vi "Main.vi"(11 "Module Admin":refnum<class "Delacor_lib_QMH_Cloneable Module Admin.lvclass">) -> ()   [LabVIEW 2020, in "TCP_Client.lvlib"]
doc: "This template is based off of the Queued Message Handler design pattern and the Queued Message Handler project template that ships with LabVIEW.\n\nThe main difference is that the queue is private to this module and communication between modules is performed via Broadcast and Request events.\n\nRequest events are wrapped in public API methods and are handled in the Event Handling Loop (EHL) of this VI. Any module can register for Broadcast events sent by this module. The EHL generates messages based on user interface actions.\n\nThe Message Handling Loop (MHL) processes messages generated by the EHL, or by other messages. The messages are string values, so new messages can be added easily to the Message Cases case structure in the MHL. Each message cluster can also provide an optional value for Message Data, which is a variant that can be converted to whatever message-specific data is required.\n_____\nBased on DQMH Project Template 6.0.0.91."
uses:
  TCP_Client.lvlib
  <vilib>/Delacor/Delacor QMH/Libraries/Cloneable Module Admin_class/Delacor_lib_QMH_Cloneable Module Admin.lvclass
  C:/Program Files (x86)/National Instruments/LabVIEW 2020/vi.lib/Delacor/Delacor QMH/Libraries/Module Admin_class/Delacor_lib_QMH_Module Admin.lvclass
  Module Data--cluster.ctl
  <vilib>/Delacor/Delacor QMH/Libraries/Cloneable Module Admin_class/Delacor_lib_QMH_Cloneable Module Admin.lvclass/Delacor_lib_QMH_Cloneable Module Admin.ctl
  <vilib>/Delacor/Delacor QMH/Libraries/Message Queue_class/Delacor_lib_QMH_Message Queue.lvclass/Delacor_lib_QMH_Message Queue.ctl
  Stop Argument--cluster.ctl
  <vilib>/Delacor/Delacor QMH/Libraries/Module Admin_class/Delacor_lib_QMH_Module Admin.lvclass/Delacor_lib_QMH_Module Admin.ctl
  <vilib>/Utility/miscctls.llb/LVPointTypeDef.ctl
  <vilib>/Delacor/Delacor QMH/Libraries/Cloneable Module Admin_class/Delacor_lib_QMH_Get Module ID.vi
  <vilib>/Delacor/Delacor QMH/Libraries/Message Queue_class/Delacor_lib_QMH_Enqueue Message (Single).vi
  <vilib>/Delacor/Delacor QMH/Libraries/Module Admin_class/Delacor_lib_QMH_Get External Launch.vi
  <vilib>/Utility/error.llb/Error Cluster From Error Code.vi
  <vilib>/ErrorRing/Error Ring.xnode
  <vilib>/Delacor/Delacor QMH/Libraries/Message Queue_class/Delacor_lib_QMH_Message Queue.lvclass
  TCP_Server/TCP_Server.lvlib
panel:
  out "Module ID":i32=-1
  out "Receive":T1 {"Horizontal Pointer Slide" scale=0.0..10.0; "Gauge" scale=0.0..10.0}
  out "Data from Server":dbl(graph)
  out "error out":errorcluster
  out "Status":string
  in  "Simulate EHL Error":bool
  in  "Simulate MHL Error":bool
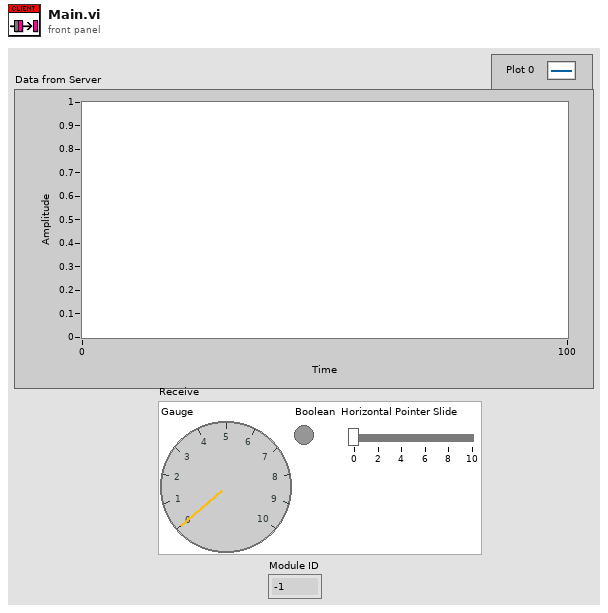
[diagram p1: front panel]
types:
  T1 = cluster{"Gauge":dbl, "Boolean":bool, "Horizontal Pointer Slide":i32}
  T2 = typedef "TCP_Client.lvlib/Request Events--cluster.ctl" = cluster{"Stop Module":refnum<user-event>, "Show Panel":refnum<user-event>, "Hide Panel":refnum<user-event>, "Show Diagram":refnum<user-event>, "Get Module Execution Status":refnum<user-event>, "Connect TCP to Server":refnum<user-event>, "CheckClientSelection":refnum<user-event>, "AllSelection":refnum<user-event>}
  T3 = typedef "TCP_Server.lvlib/Broadcast Events--cluster.ctl" = cluster{"Module Did Init":refnum<user-event>, "Status Updated":refnum<user-event>, "Error Reported":refnum<user-event>, "Module Did Stop":refnum<user-event>, "Update Module Execution Status":refnum<user-event>, "ClientSelect":refnum<user-event>, "SelectAll":refnum<user-event>}
  T4 = typedef "TCP_Client.lvlib/Module Data--cluster.ctl" = cluster{"Status":string}
  T5 = cluster{"Gauge":dbl, "Boolean":bool, "Horizontal Pointer Slide":dbl}
  T6 = enum32{"invalid lock state", "Not Locked", "Locked (No Password)", "Password-protected"}
  T7 = typedef "TCP_Client.lvlib/Stop Argument--cluster.ctl" = cluster{"Module ID":i32, "Origin":string, "Exit via Stop Module Req?":bool, "Wait for Module to stop?":bool}
  T8 = typedef "LVPointTypeDef.ctl" = cluster{"Horizontal":i16, "Vertical":i16}
  T9 = enum32{"Invalid", "Standard", "Closed", "Hidden", "Minimized", "Maximized"}
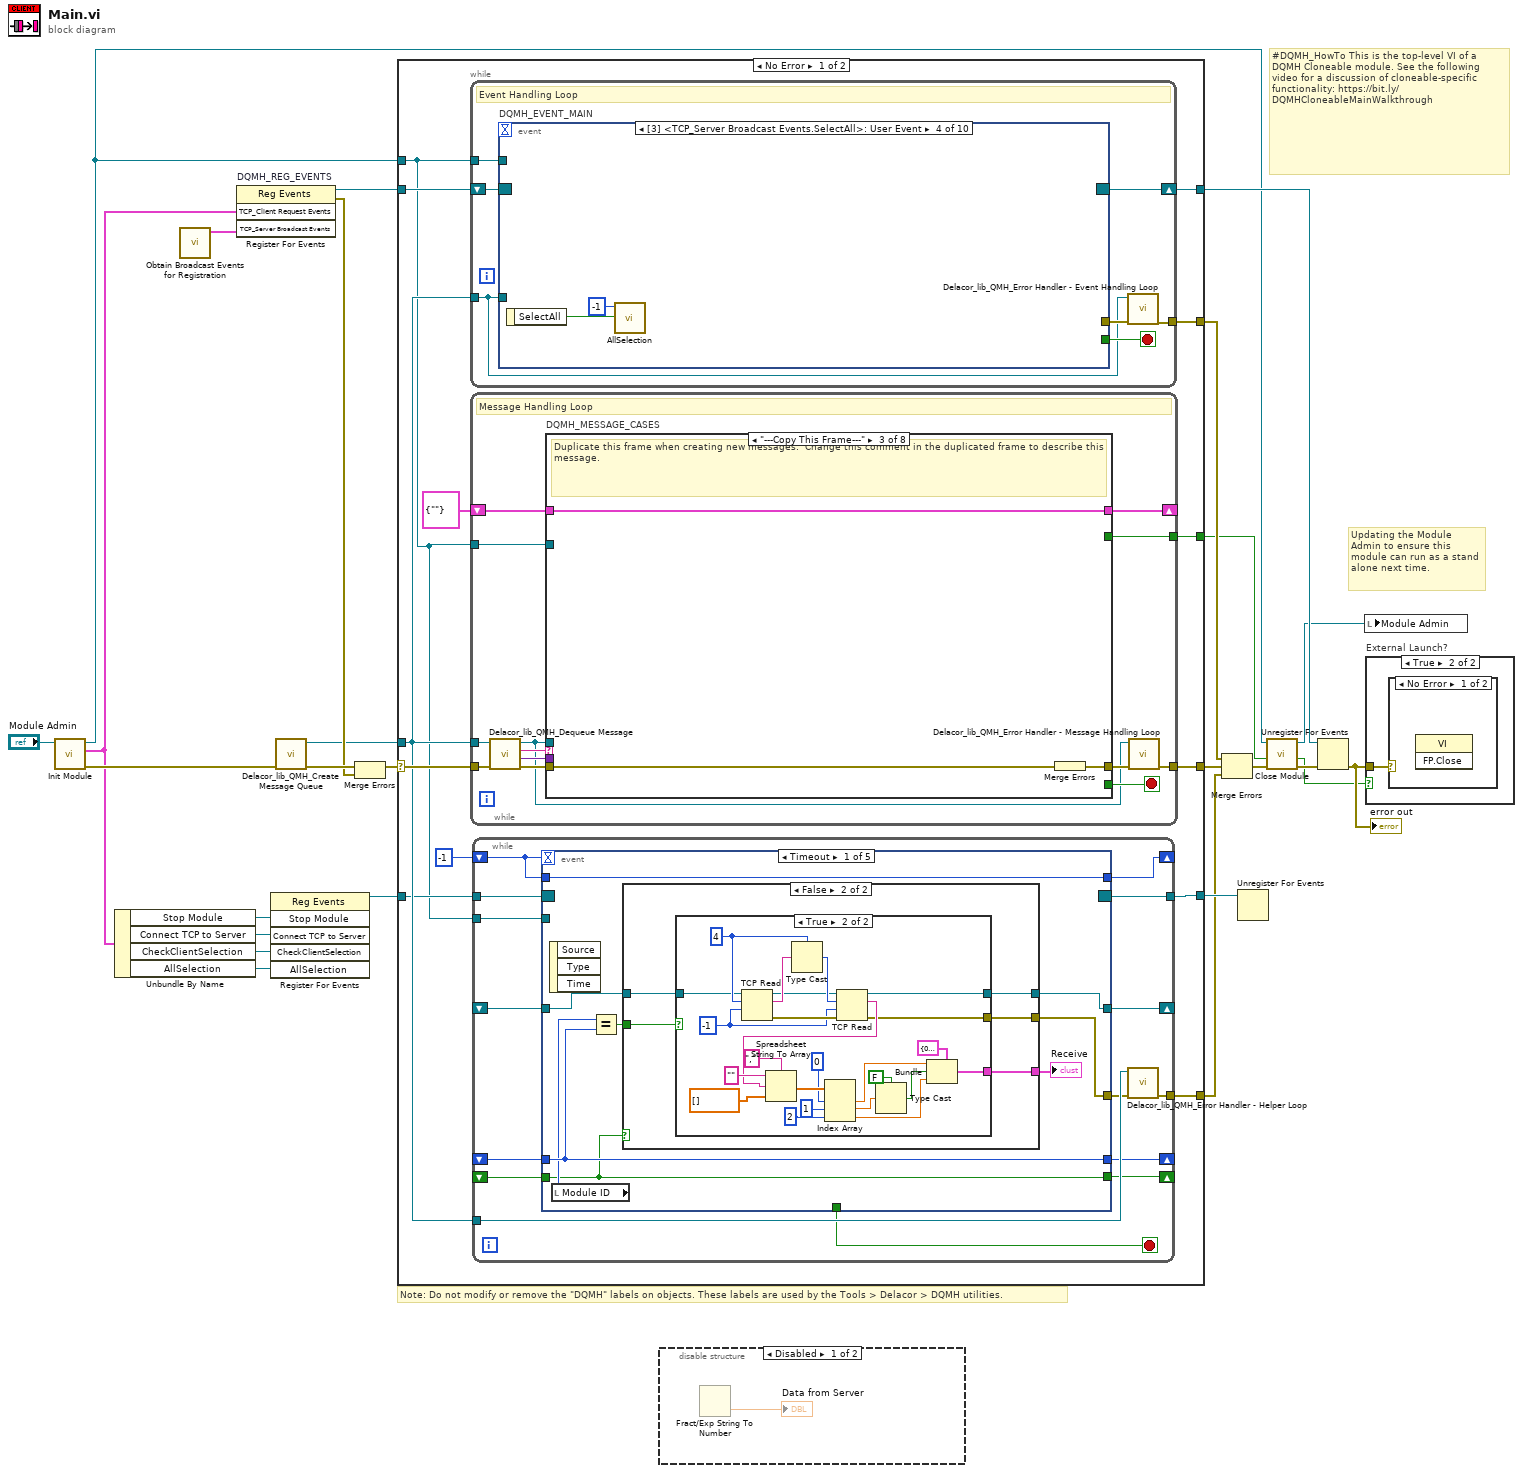
[diagram p0: block diagram]
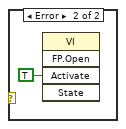
[diagram p4: hidden frame]
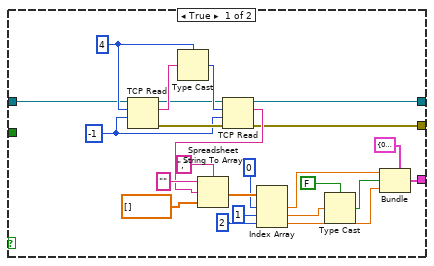
[diagram p5: hidden frame]
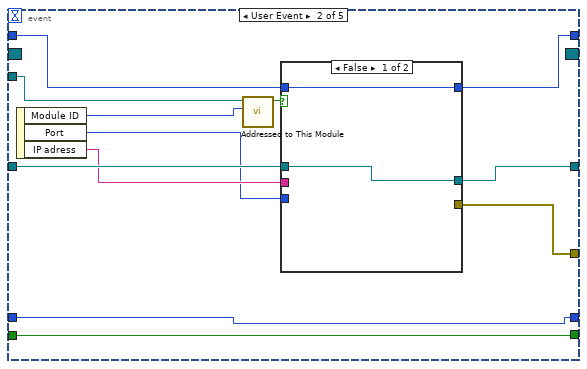
[diagram p7: hidden frame]
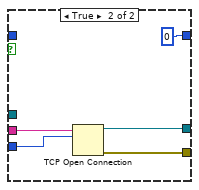
[diagram p8: hidden frame]
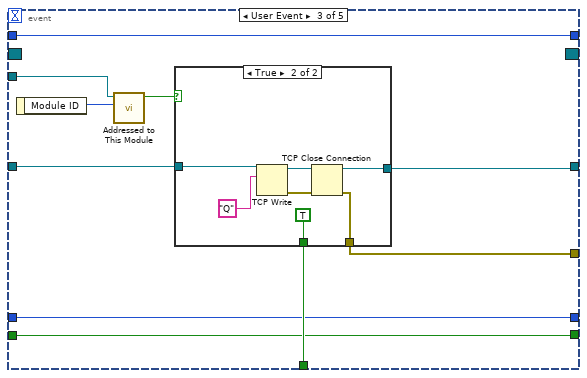
[diagram p9: hidden frame]
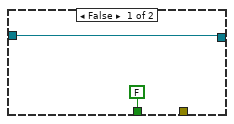
[diagram p10: hidden frame]
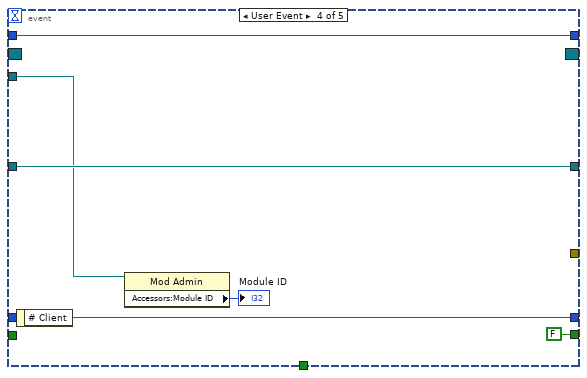
[diagram p11: hidden frame]
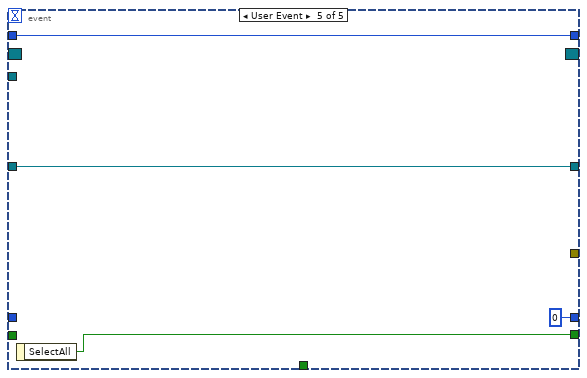
[diagram p12: hidden frame]
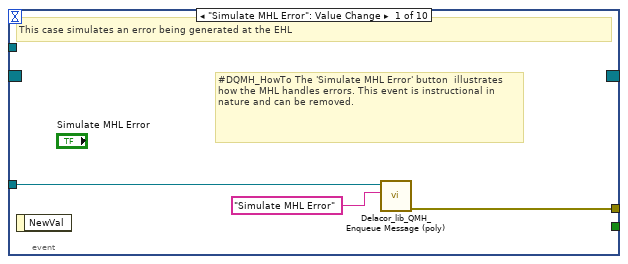
[diagram p13: hidden frame]
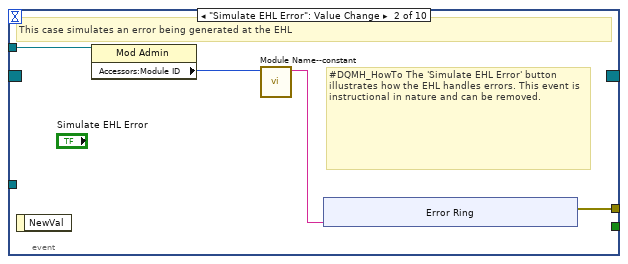
[diagram p14: hidden frame]
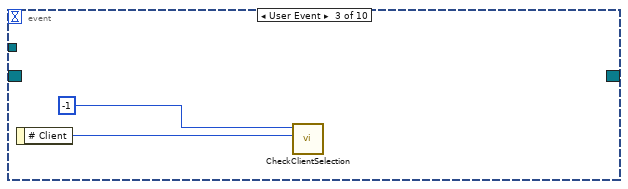
[diagram p15: hidden frame]
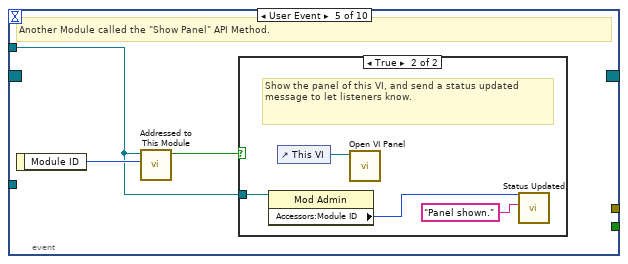
[diagram p16: hidden frame]
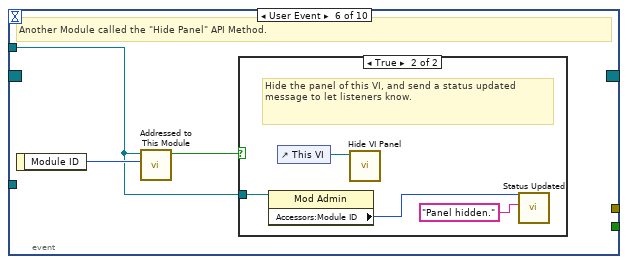
[diagram p18: hidden frame]
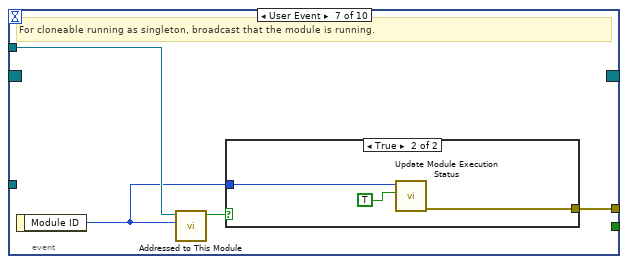
[diagram p20: hidden frame]
diagram:
  # "#DQMH_HowTo This is the top-level VI of a DQMH Cloneable module. See the following video for a discussion of cloneable-specific functionality: https://bit.ly/DQMHCloneableMainWalkthrough"
  # "Note: Do not modify or remove the \"DQMH\" labels on objects. These labels are used by the Tools > Delacor > DQMH utilities."
  # "Updating the Module Admin to ensure this module can run as a stand alone next time."
  n1 = call "Init Module.vi"("Cloneable Module Admin in"="Module Admin") -> ("error out"=w23:errorcluster, "TCP_Client Request Events"=w7:T2, "Cloneable Module Admin out"=w13:refnum<class "Delacor_lib_QMH_Cloneable Module Admin.lvclass">)  [unwired: 8 in]
  n2 = Unbundle By Name(w7) -> ("Stop Module"=w6:refnum<user-event>, "Connect TCP to Server"=w4:refnum<user-event>, "CheckClientSelection"=w2:refnum<user-event>, "AllSelection"=w1:refnum<user-event>)
  n3 = call "Obtain Broadcast Events for Registration.vi"() -> ("TCP_Server Broadcast Events"=w3:T3)  [unwired: 9 in, 2 out]
  n4 = register-events "DQMH_REG_EVENTS"(w7, w3) -> (reference out=w16:refnum<event-registration>, error out=w18:errorcluster)  [unwired: 2 in]
  n5 = register-events(w6, w4, w2, w1) -> (reference out=w5:refnum<event-registration>)  [unwired: 2 in, 1 out]
  n6 = call <vilib>:"Delacor_lib_QMH_Create Message Queue.vi"("error in"=w23) -> ("error out"=w20:errorcluster, "Message Queue"=w15:refnum<class "Delacor_lib_QMH_Message Queue.lvclass">)  [unwired: 9 in]
  n7 = Merge Errors(w20, w18) -> (w19:errorcluster)
  n8 = case shown="No Error" w19 {
    selector: w19 -> [w37 w365]
    tunnel: [w39 w364] -> w24
    tunnel: [w36 w372] -> w17
    tunnel: w16 -> [w34 w372]
    tunnel: w15 -> [w32 w363]
    tunnel: [w38 _] -> w25
    tunnel: w13 -> [w27 w368]
    tunnel: [w33 _] -> w11
    tunnel: [w31 _] -> w9
    tunnel: [w30 _] -> w8
    tunnel: w5 -> [w29 _]
    frame No Error {
      n9 = while {
        tunnel: w32 -> [w166]
        shift-right: [w169] -> w36
        shift-left: w34 -> [w170]
        tunnel: [w171] -> w38
        tunnel: w27 -> [w167]
        stop <- w168 stop-if-true
        # "Event Handling Loop"
        n10 = event "DQMH_EVENT_MAIN" shown="[3] <TCP_Server Broadcast Events.SelectAll>: User Event" {
          selector: w170 -> [_ _ _ _ _ _ _ _ _ _]
          dyn-events: [_ _ _ _ _ _ _ _ _ _] -> w169
          timeout: _ -> [_ _ _ _ _ _ _ _ _ _]
          tunnel: [_ _ _ _ _ _ _ _ w231 _] -> w168
          tunnel: w166 -> [w174 _ _ _ _ _ _ _ w234 w250]
          tunnel: [w175 w179 _ _ _ _ w208 _ w235 w253] -> w172
          tunnel: w167 -> [_ w178 _ _ w191 w198 w206 w212 w233 w251]
          event "Simulate MHL Error": Value Change {
            # "#DQMH_HowTo The 'Simulate MHL Error' button  illustrates how the MHL handles errors. This event is instructional in nature and can be removed."
            # "This case simulates an error being generated at the EHL"
            n11 = event-data() -> ()  [unwired: 1 in, 1 out]
            n12 = call-poly <vilib>:"Delacor_lib_QMH_Enqueue Message (poly).vi"("Message"="Simulate MHL Error", "Message Queue in"=w174) -> ("error out"=w175:errorcluster)  [unwired: 8 in, 1 out]
          }
          event "Simulate EHL Error": Value Change {
            # "#DQMH_HowTo The 'Simulate EHL Error' button  illustrates how the EHL handles errors. This event is instructional in nature and can be removed."
            # "This case simulates an error being generated at the EHL"
            n13 = event-data() -> ()  [unwired: 1 in, 1 out]
            n14 = property class="Mod Admin"(reference=w178) -> ("Accessors:Module ID"=w177:i32)  [unwired: 1 in, 2 out]
            n15 = call "Module Name--constant.vi"("Module ID"=w177) -> ("Module Name"=w176:string)  [unwired: 10 in]
            n16 = xnode "Error Ring"("parameter 0"=w176) -> ("error out"=w179:errorcluster)
          }
          event User Event {
            n17 = event-data() -> ("# Client"=w188:i32)  [unwired: 1 in]
            n18 = call "CheckClientSelection.vi"("# Client"=w188, "Module ID"=-1) -> ()  [unwired: 9 in, 1 out]
          }
          event User Event {
            n19 = event-data() -> ("SelectAll"=w190:bool)  [unwired: 1 in]
            n20 = call "AllSelection.vi"("SelectAll"=w190, "Module ID"=-1) -> ()  [unwired: 9 in, 1 out]
          }
          event User Event {
            # "Another Module called the \"Show Panel\" API Method."
            n21 = event-data() -> ("Module ID"=w192:i32)  [unwired: 1 in]
            n22 = call "Addressed to This Module.vi"("Module ID from Argument"=w192, "Module Admin"=w191) -> ("Addressed to this instance?"=w193:bool)  [unwired: 8 in, 1 out]
            n23 = case shown="True" w193 {
              tunnel: w191 -> [_ w195]
              frame False {
              }
              frame True {
                # "Show the panel of this VI, and send a status updated message to let listeners know."
                n24 = property class="Mod Admin"(reference=w195) -> ("Accessors:Module ID"=w194:i32)  [unwired: 1 in, 2 out]
                n25 = control-ref of="This VI"() -> (w197:refnum<vi>)
                n26 = call "Open VI Panel.vi"("VI"=w197) -> ()  [unwired: 10 in, 1 out]
                n27 = call "Status Updated.vi"("Status"="Panel shown." ("format string"), "Module ID"=w194) -> ()  [unwired: 9 in, 1 out]
              }
            }
          }
          event User Event {
            # "Another Module called the \"Hide Panel\" API Method."
            n28 = event-data() -> ("Module ID"=w199:i32)  [unwired: 1 in]
            n29 = call "Addressed to This Module.vi"("Module ID from Argument"=w199, "Module Admin"=w198) -> ("Addressed to this instance?"=w200:bool)  [unwired: 8 in, 1 out]
            n30 = case shown="True" w200 {
              tunnel: w198 -> [_ w202]
              frame False {
              }
              frame True {
                # "Hide the panel of this VI, and send a status updated message to let listeners know."
                n31 = property class="Mod Admin"(reference=w202) -> ("Accessors:Module ID"=w201:i32)  [unwired: 1 in, 2 out]
                n32 = control-ref of="This VI"() -> (w204:refnum<vi>)
                n33 = call "Hide VI Panel.vi"("VI"=w204) -> ()  [unwired: 10 in, 1 out]
                n34 = call "Status Updated.vi"("Status"="Panel hidden." ("format string"), "Module ID"=w201) -> ()  [unwired: 9 in, 1 out]
              }
            }
          }
          event User Event {
            # "For cloneable running as singleton, broadcast that the module is running."
            n35 = event-data() -> ("Module ID"=w205:i32)  [unwired: 1 in]
            n36 = call "Addressed to This Module.vi"("Module ID from Argument"=w205, "Module Admin"=w206) -> ("Addressed to this instance?"=w207:bool)  [unwired: 8 in, 1 out]
            n37 = case shown="True" w207 {
              tunnel: [_ w211] -> w208
              tunnel: w205 -> [_ w210]
              frame False {
              }
              frame True {
                n38 = call "Update Module Execution Status.vi"("Running?"=TRUE, "Module ID"=w210) -> ("error out"=w211:errorcluster)  [unwired: 9 in]
              }
            }
          }
          event User Event {
            # "Another Module called the \"Show Diagram\" API Method. This event is used for debugging."
            n39 = event-data() -> ("Module ID"=w213:i32)  [unwired: 1 in]
            n40 = call "Addressed to This Module.vi"("Module ID from Argument"=w213, "Module Admin"=w212) -> ("Addressed to this instance?"=w214:bool)  [unwired: 8 in, 1 out]
            n41 = case shown="True" w214 {
              tunnel: w212 -> [_ w215]
              frame False {
              }
              frame True {
                n42 = disable-structure shown="RUN_TIME_ENGINE==False" {
                  disable-tunnel: w215 -> [w216 _]
                  frame condition #0 (active) {
                    # "functionality not available in exe"
                    n43 = invoke class="VI" method="Lock State.Get"() -> (error out=w222:errorcluster, "Get Lock State"=w221:T6, "pwd in cache"=w218:bool)  [unwired: 4 in, 1 out]
                    n44 = Equal?(x=T6."Password-protected", y=w221) -> (x = y?=w219:bool)
                    n45 = Compound Arithmetic op=AND(w219, invert w218) -> (w217:bool)
                    n46 = case shown="False" w217 {
                      tunnel: w222 -> [w227 _]
                      tunnel: w216 -> [w224 _]
                      frame False {
                        n47 = property class="Mod Admin"(reference=w224) -> ("Accessors:Module ID"=w223:i32)  [unwired: 1 in, 2 out]
                        n48 = property class="VI"(error in=w227, "BDWin.Open"=TRUE ("Block Diagram Window:Open")) -> ()  [unwired: 1 in, 2 out]
                        n49 = call "Status Updated.vi"("Status"="Block Diagram shown." ("format string"), "Module ID"=w223) -> ()  [unwired: 9 in, 1 out]
                      }
                      frame True {
                        # "Password-protected VI, and the password is not in the cache. Do not show the diagram."
                      }
                    }
                  }
                  frame condition #1 {
                  }
                }
              }
            }
          }
          event User Event {
            # "Another Module called the \"Stop Module\" API Method  or the Message Handling Loop below."
            n50 = event-data() -> ("Module ID"=w229:i32, "Wait for Module to stop?"=w230:bool, "Origin"=w228:string)  [unwired: 1 in]
            n51 = call "Addressed to This Module.vi"("Module ID from Argument"=w229, "Module Admin"=w233) -> ("Addressed to this instance?"=w232:bool)  [unwired: 8 in, 1 out]
            n52 = case shown="True" w232 {
              tunnel: [_ w247] -> w235
              tunnel: w234 -> [_ w243]
              tunnel: [_ TRUE] -> w231
              tunnel: w230 -> [_ w238]
              tunnel: w229 -> [_ w240]
              tunnel: w228 -> [_ w236]
              frame False {
              }
              frame True {
                # "The event can get fired from the Exit message. The queue gets destroyed there. In this case, the Enqueue VI will return error 1. It is safe to ignore, because the module is already exiting."
                n53 = local write "Status"(w236) -> ()
                n54 = Bundle By Name(cluster=T7 {"Module ID"=-1, "Origin"="", "Exit via Stop Module Req?"=FALSE, "Wait for Module to stop?"=FALSE} ("Stop Argument"), "Module ID"=w240, "Exit via Stop Module Req?"=TRUE, "Wait for Module to stop?"=w238) -> (w237:T7)
                n55 = call-poly <vilib>:"Delacor_lib_QMH_Enqueue Message (poly).vi"("Priority Message? (F)"=TRUE, "Message Data"=w237, "Message"="Exit", "Message Queue in"=w243) -> ("error out"=w248:errorcluster)  [unwired: 6 in, 1 out]
                n56 = call <vilib>:"Clear Errors.vi"("error in (no error)"=w248, "specific error code to clear (0: all)"=1) -> ("error out"=w247:errorcluster)  [unwired: 4 in, 1 out]
              }
            }
          }
          event Panel Close? {
            w252 = TRUE  # Discard the event, the MHL is responsible for closing and stopping this VI.
            # "Hide the panel or send the 'Exit' message if the user clicks the 'X' on the module main VI panel."
            n57 = event-data() -> ()  [unwired: 1 in, 1 out]
            n58 = property class="Mod Admin"(reference=w251) -> ("Accessors:External Launch"=w249:bool)  [unwired: 1 in, 2 out]
            n59 = case shown="True" w249 {
              tunnel: w250 -> [_ w257]
              tunnel: [_ w258] -> w253
              frame True {
                # "If externally launched, clicking the 'X' hides the panel, but doesn't close it."
                n60 = control-ref of="This VI"() -> (w254:refnum<vi>)
                n61 = call "Hide VI Panel.vi"("VI"=w254) -> ()  [unwired: 10 in, 1 out]
              }
              frame False {
                # "If run as a stand-alone VI, clicking the panel 'X' stops the VI."
                n62 = call-poly <vilib>:"Delacor_lib_QMH_Enqueue Message (poly).vi"("Priority Message? (F)"=TRUE, "Message"="Exit", "Message Queue in"=w257) -> ("error out"=w258:errorcluster)  [unwired: 7 in, 1 out]
              }
            }
            n63 = event-data("Discard?"=w252) -> ()  [unwired: 1 in, 1 out]
          }
        }
        n64 = call-dynamic "Delacor_lib_QMH_Error Handler - Event Handling Loop.vi"("error in"=w172, "Message Queue in"=w166) -> ("dup error in"=w171:errorcluster)  [unwired: 8 in, 1 out]
      }
      n65 = while {
        tunnel: w32 -> [w262]
        shift-right: [w266] -> _
        shift-left: T4 {"Status"=""} ("Data Cluster") -> [w267]
        tunnel: w37 -> [w270]
        tunnel: [w268] -> w39
        tunnel: w27 -> [w260]
        tunnel: [w259] -> w33
        stop <- w265 stop-if-true
        # "Message Handling Loop"
        n66 = call-dynamic "Delacor_lib_QMH_Dequeue Message.vi"("error in"=w270, "Message Queue in"=w262) -> ("error out"=w269:errorcluster, "Message Data"=w263:variant, "Message"=w264:string, "Message Queue out"=w261:refnum<class "Delacor_lib_QMH_Message Queue.lvclass">)  [unwired: 6 in]
        n67 = case "DQMH_MESSAGE_CASES" shown="\"---Copy This Frame---\"" w264 {
          selector: w264 -> [_ _ _ _ _ _ _ w350]
          tunnel: w261 -> [_ _ _ _ w301 _ w340 _]
          tunnel: w269 -> [w290 w294 w297 w299 w310 w323 w346 w352]
          tunnel: [w288 w294 w296 w299 w306 w322 w343 w353] -> w271
          tunnel: w267 -> [w281 w293 w295 w298 w305 w320 w339 w351]
          tunnel: [w280 w293 w295 w298 w305 w320 w339 w351] -> w266
          tunnel: [_ _ _ _ _ _ w338 _] -> w265
          tunnel: w263 -> [_ _ _ _ w304 _ w336 _]
          tunnel: w260 -> [w275 _ _ _ w303 w318 w332 w348]
          tunnel: [_ _ _ _ _ _ w334 _] -> w259
          frame "Initialize" {
            w272 = "Initial Message" ("Initial Message")
            # "#CodeNeeded - Initialize the appearance of the front panel."
            # "#CodeNeeded - Initialize your state data here."
            # "Initialize - Any operation that needs to be done before the module can receive messages. Synchronize Caller Events.vi will inform Start Module.vi that the module has launched and is ready to receive messages. Module Did Init.vi will broadcast that the module initialized."
            n68 = call "Synchronize Caller Events.vi"("error in (no error)"=w290, "Module Admin"=w275) -> ("error out"=w289:errorcluster, "Module Admin out"=w274:refnum<class "Delacor_lib_QMH_Cloneable Module Admin.lvclass">)  [unwired: 8 in]
            n69 = property class="Mod Admin"(reference=w274) -> ("Accessors:Module ID"=w277:i32, "Accessors:External Launch"=w276:bool)  [unwired: 1 in, 2 out]
            n70 = call "Module Name--constant.vi"("Module ID"=w277) -> ("Module Name"=w285:string)  [unwired: 10 in]
            n71 = property class="VI"("Front Panel.Title"=w285) -> (reference out=w287:refnum<vi>, error out=w292:errorcluster)  [unwired: 2 in]
            n72 = Select(t=T9."Hidden" ("State"), s=w276, f=T9."Standard" ("State")) -> (s? t:f=w282:T9)
            n73 = invoke class="VI" method="FP.Open"(reference=w287, error in=w292, "State"=w282) -> (reference out=w286:refnum<vi>, error out=w291:errorcluster)  [unwired: 2 in, 3 out]
            n74 = call "Module Name--constant.vi"("Module ID"=w277) -> ("Module Name"=w278:string)  [unwired: 10 in]
            n75 = Bundle By Name(cluster=w281, "Status"=w272) -> (w280:T4)
            n76 = invoke class="VI" method="FP.Center"(reference=w286, error in=w291) -> ()  [unwired: 1 in, 3 out]
            n77 = property on="Pane" class="Pane"("Origin"=T8 {"Horizontal"=0, "Vertical"=0}) -> ()  [unwired: 2 in, 2 out]
            n78 = call "Module Did Init.vi"("error in (no error)"=w289, "Initialized?"=TRUE, "Origin"=w278, "Module ID"=w277) -> ("error out"=w288:errorcluster)  [unwired: 7 in]
            "Status" <- w272
          }
          frame "---Module Specific---" {
            # "Separator -- The following cases handle messages specific to this Module."
          }
          frame "---Copy This Frame---" {
            # "Duplicate this frame when creating new messages.  Change this comment in the duplicated frame to describe this message."
            n79 = Merge Errors(w297) -> (w296:errorcluster)
          }
          frame "---Exit and Error Handling---" {
            # "Separator - the following cases handle errors and exit messages."
          }
          frame "Error" {
            # "#CodeRecommended - If you ever change the name of this \"Error\" message, you'll need to update the name in the Check Loop Error.vi as well."
            # "#CodeRecommended - If the module is running in standalone mode (External Launch = FALSE), this code will pop up an error dialog and call the 'Exit' message if an error occurs. Add more fine-grained error handling here."
            # "Error - Check the error message data and respond accordingly. This message is sent by the \"Error Handler\" VIs at the end of each loop in this application."
            n80 = property class="Mod Admin"(reference=w303) -> ("Accessors:External Launch"=w302:bool, "Accessors:Module ID"=w300:i32)  [unwired: 1 in, 2 out]
            n81 = Variant To Data(error in=w310, type=errorcluster {"status"=FALSE, "code"=0, "source"=""} ("error constant"), Variant=w304) -> (data=w311:errorcluster, error out=w308:errorcluster)
            n82 = call "Error Reported.vi"("Error"=w311, "Module ID"=w300) -> ()  [unwired: 9 in, 1 out]
            n83 = case shown="False" w302 {
              tunnel: [w316 _] -> w307
              tunnel: w301 -> [w314 _]
              tunnel: w311 -> [w315 _]
              frame False {
                # "If the module is running standalone, then pop up an error dialog and call the \"Exit\" message."
                n84 = call <vilib>:"Simple Error Handler.vi"("error in (no error)"=w315) -> ()  [unwired: 4 in, 5 out]
                n85 = call-poly <vilib>:"Delacor_lib_QMH_Enqueue Message (poly).vi"("Priority Message? (F)"=TRUE, "Message"="Exit", "Message Queue in"=w314) -> ("error out"=w316:errorcluster)  [unwired: 7 in, 1 out]
              }
              frame True {
                # "If the module was launched externally, calling the Error Reported broadcast VI is the only action performed by the \"Error\" message. The module's caller can then process the error appropriately."
              }
            }
            n86 = Merge Errors(w308, w307) -> (w306:errorcluster)
            n87 = local write "error out"(w306) -> ()
          }
          frame "Simulate MHL Error" {
            # "#DQMH_HowTo The 'Simulate MHL Error' button  illustrates how the MHL handles errors. This event is instructional in nature and can be removed."
            # "Simulate an error occurring at the MHL"
            n88 = property class="Mod Admin"(reference=w318) -> ("Accessors:Module ID"=w319:i32)  [unwired: 1 in, 2 out]
            n89 = call "Module Name--constant.vi"("Module ID"=w319) -> ("Module Name"=w317:string)  [unwired: 10 in]
            n90 = xnode "Error Ring"("parameter 0"=w317) -> ("error out"=w321:errorcluster)
            n91 = Merge Errors(w323, w321) -> (w322:errorcluster)
          }
          frame "Exit" {
            w337 = 91  # 91: not all Exit messages will have an argument
            w338 = TRUE  # Stop the VI
            # "Release the message queue reference"
            # "#CodeNeeded - Add any required cleanup code here."
            # "Exit - Exit the application."
            n92 = Variant To Data(error in=w346, type=T7 {"Module ID"=-1, "Origin"="", "Exit via Stop Module Req?"=FALSE, "Wait for Module to stop?"=FALSE} ("Stop Argument"), Variant=w336) -> (data=w333:T7, error out=w341:errorcluster)
            n93 = call <vilib>:"Clear Errors.vi"("error in (no error)"=w341, "specific error code to clear (0: all)"=w337) -> ("error out"=w345:errorcluster)  [unwired: 4 in, 1 out]
            n94 = control-ref of="This VI"() -> (w331:refnum<vi>)
            n95 = call-dynamic "Delacor_lib_QMH_Release Message Queue.vi"("error in"=w345, "Message Queue"=w340) -> ("error out"=w344:errorcluster)  [unwired: 9 in]
            n96 = call "Handle Exit.vi"("Stop Argument"=w333, "Module Admin in"=w332, "VI reference"=w331) -> ("error out"=w342:errorcluster, "Wait for Stop?"=w334:bool)  [unwired: 7 in]
            n97 = Merge Errors(w344, w342) -> (w343:errorcluster)
          }
          frame Default {
            # "'Default' case only runs if there is a message that isn't defined in any of the other cases.  Output a programming error."
            n98 = property class="Mod Admin"(reference=w348) -> ("Accessors:Module ID"=w347:i32)  [unwired: 1 in, 2 out]
            n99 = call "Module Name--constant.vi"("Module ID"=w347) -> ("Module Name"=w349:string)  [unwired: 10 in]
            n100 = xnode "Error Ring"("parameter 0"=w350, "parameter 1"=w349) -> ("error out"=w354:errorcluster)
            n101 = Merge Errors(w352, w354) -> (w353:errorcluster)
          }
        }
        n102 = call-dynamic "Delacor_lib_QMH_Error Handler - Message Handling Loop.vi"("error in"=w271, "Message Queue in"=w261) -> ("dup error in"=w268:errorcluster)  [unwired: 8 in, 1 out]
      }
      n103 = while {
        tunnel: w32 -> [w54]
        tunnel: [w53] -> w31
        tunnel: [w52] -> w30
        tunnel: w29 -> [w51]
        shift-right: [w49] -> _
        shift-left: -1 -> [w50]
        shift-right: [w46] -> _
        shift-left: _ -> [w47]
        tunnel: w27 -> [w44]
        shift-right: [w43] -> _
        shift-left: _ -> [w41]
        shift-right: [w42] -> _
        shift-left: _ -> [w40]
        stop <- w48 stop-if-true
        n104 = event shown="[0] Timeout" {
          selector: w51 -> [_ _ _ _ _]
          dyn-events: [_ _ _ _ _] -> w53
          timeout: w50 -> [_ _ _ _ _]
          tunnel: w50 -> [w63 w125 w146 w159 w164]
          tunnel: [w63 w124 w146 w159 w164] -> w49
          tunnel: [_ _ w145 _ _] -> w48
          tunnel: w47 -> [w62 w129 w144 w160 w163]
          tunnel: [w61 w128 w143 w160 w163] -> w46
          tunnel: [w60 w121 w142 _ _] -> w45
          tunnel: w44 -> [_ w122 w141 w158 _]
          tunnel: [w59 w120 w137 w161 0 ("# Client")] -> w43
          tunnel: [w57 w118 w138 FALSE ("SelectAll") w165] -> w42
          tunnel: w41 -> [w59 w120 w137 _ _]
          tunnel: w40 -> [w57 w118 w138 _ _]
          event Timeout {
            n105 = event-data() -> ()  [unwired: 1 in, 3 out]
            n106 = local read "Module ID"() -> (w58:i32)
            n107 = Equal?(x=w58, y=w59) -> (x = y?=w55:bool)
            n108 = case shown="False" w57 {
              tunnel: w62 -> [w81 w92]
              tunnel: [w80 w91] -> w61
              tunnel: [w66 w90] -> w60
              tunnel: [w64 w89] -> w56
              tunnel: w55 -> [_ w88]
              frame True {
                w82 = -1
                w83 = 4
                n109 = TCP Read(connection ID=w81, bytes to read=w83, 9:w82) -> (connection ID out=w84:refnum<k5>, data out=w87:string, error out=w86:errorcluster)  [unwired: 1 in, 1 out]
                n110 = Type Cast(type=w83, x=w87) -> (*(type *) &x=w85:i32)
                n111 = TCP Read(connection ID=w84, bytes to read=w85, error in (no error)=w86, 9:w82) -> (connection ID out=w80:refnum<k5>, data out=w67:string, error out=w66:errorcluster)  [unwired: 1 out]
                n112 = Spreadsheet String To Array(delimiter (Tab)=",", format string="", spreadsheet string=w67, array type (2D Dbl)=dbl[] []) -> (array=w79:dbl[])
                n113 = Index Array(array=w79, index #1=0 ("index"), index #2=1 ("index"), index #3=2 ("index")) -> (element #1=w78:dbl, element #2=w76:dbl, element #3=w77:dbl)
                n114 = Type Cast(type=FALSE, x=w76) -> (*(type *) &x=w75:bool)
                n115 = Bundle(cluster=T5 {"Gauge"=0.0, "Boolean"=FALSE, "Horizontal Pointer Slide"=5.0} ("Receive"), "Gauge"=w78, "Boolean"=w75, "Horizontal Pointer Slide"=w77) -> (w64:T5)
              }
              frame False {
                n116 = case shown="True" w88 {
                  tunnel: w92 -> [w93 w111]
                  tunnel: [w93 w110] -> w91
                  tunnel: [_ w96] -> w90
                  tunnel: [_ w94] -> w89
                  frame False {
                  }
                  frame True {
                    w112 = -1
                    w113 = 4
                    n117 = TCP Read(connection ID=w111, bytes to read=w113, 9:w112) -> (connection ID out=w114:refnum<k5>, data out=w117:string, error out=w116:errorcluster)  [unwired: 1 in, 1 out]
                    n118 = Type Cast(type=w113, x=w117) -> (*(type *) &x=w115:i32)
                    n119 = TCP Read(connection ID=w114, bytes to read=w115, error in (no error)=w116, 9:w112) -> (connection ID out=w110:refnum<k5>, data out=w97:string, error out=w96:errorcluster)  [unwired: 1 out]
                    n120 = Spreadsheet String To Array(delimiter (Tab)=",", format string="", spreadsheet string=w97, array type (2D Dbl)=dbl[] []) -> (array=w109:dbl[])
                    n121 = Index Array(array=w109, index #1=0 ("index"), index #2=1 ("index"), index #3=2 ("index")) -> (element #1=w108:dbl, element #2=w106:dbl, element #3=w107:dbl)
                    n122 = Type Cast(type=FALSE, x=w106) -> (*(type *) &x=w105:bool)
                    n123 = Bundle(cluster=T5 {"Gauge"=0.0, "Boolean"=FALSE, "Horizontal Pointer Slide"=5.0} ("Receive"), "Gauge"=w108, "Boolean"=w105, "Horizontal Pointer Slide"=w107) -> (w94:T5)
                  }
                }
              }
            }
            "Receive" <- w56
          }
          event User Event {
            n124 = event-data() -> ("Module ID"=w123:i32, "Port"=w126:u16, "IP adress"=w127:string)  [unwired: 1 in]
            n125 = call "Addressed to This Module.vi"("Module ID from Argument"=w123, "Module Admin"=w122) -> ("Addressed to this instance?"=w119:bool)  [unwired: 8 in, 1 out]
            n126 = case shown="False" w119 {
              tunnel: w127 -> [_ w136]
              tunnel: w126 -> [_ w135]
              tunnel: [_ w134] -> w121
              tunnel: [w131 w133] -> w128
              tunnel: w129 -> [w131 _]
              tunnel: w125 -> [w130 _]
              tunnel: [w130 0] -> w124
              frame False {
              }
              frame True {
                n127 = TCP Open Connection(address=w136, remote port or service name=w135) -> (connection ID=w133:refnum<k5>, error out=w134:errorcluster)  [unwired: 1 in, 2 out]
              }
            }
          }
          event User Event {
            n128 = event-data() -> ("Module ID"=w140:i32)  [unwired: 1 in]
            n129 = call "Addressed to This Module.vi"("Module ID from Argument"=w140, "Module Admin"=w141) -> ("Addressed to this instance?"=w139:bool)  [unwired: 8 in, 1 out]
            n130 = case shown="True" w139 {
              tunnel: [FALSE TRUE] -> w145
              tunnel: w144 -> [w148 w154]
              tunnel: [w148 w152] -> w143
              tunnel: [_ w149] -> w142
              frame False {
              }
              frame True {
                n131 = TCP Write(connection ID=w154, data in="Q") -> (connection ID out=w153:refnum<k5>, error out=w150:errorcluster)  [unwired: 1 in, 2 out]
                n132 = TCP Close Connection(connection ID=w153, error in (no error)=w150) -> (connection ID out=w152:refnum<k5>, error out=w149:errorcluster)  [unwired: 1 out]
              }
            }
          }
          event User Event {
            n133 = event-data() -> ("# Client"=w161:i32)  [unwired: 1 in]
            n134 = property class="Mod Admin"(reference=w158) -> ("Accessors:Module ID"=→"Module ID":i32)  [unwired: 1 in, 2 out]
          }
          event User Event {
            n135 = event-data() -> ("SelectAll"=w165:bool)  [unwired: 1 in]
          }
        }
        n136 = call-dynamic "Delacor_lib_QMH_Error Handler - Helper Loop.vi"("error in"=w45, "Message Queue in"=w54) -> ("dup error in"=w52:errorcluster)  [unwired: 8 in, 1 out]
      }
    }
    frame Error {
      n137 = call "Synchronize Caller Events.vi"("Module Admin"=w368) -> ("Module Admin out"=w367:refnum<class "Delacor_lib_QMH_Cloneable Module Admin.lvclass">)  [unwired: 9 in, 1 out]
      n138 = property class="Mod Admin"(reference=w367) -> ("Accessors:Module ID"=w366:i32)  [unwired: 1 in, 2 out]
      n139 = call-dynamic "Delacor_lib_QMH_Release Message Queue.vi"("error in"=w365, "Message Queue"=w363) -> ("error out"=w364:errorcluster)  [unwired: 9 in]
      n140 = call "Module Name--constant.vi"("Module ID"=w366) -> ("Module Name"=w371:string)  [unwired: 10 in]
      n141 = Format Into String(format string="An error occurred during initialization. %s is no longer running.", w371) -> (resulting string=w369:string)  [unwired: 2 in, 1 out]
      n142 = call "Error Reported.vi"("Additional Information"=w369, "Error"=w364, "Module ID"=w366) -> ()  [unwired: 8 in, 1 out]
    }
  }
  n143 = disable-structure shown="Disabled" {
    frame Disabled {
      n144 = Fract/Exp String To Number() -> (number=→"Data from Server":dbl)  [unwired: 4 in, 1 out]
    }
    frame Enabled {
    }
  }
  n145 = Merge Errors(w25, w24, w8) -> (w26:errorcluster)
  n146 = Unregister For Events(event registration refnum=w9) -> ()  [unwired: 1 in, 1 out]
  n147 = call "Close Module.vi"("error in"=w26, "Wait for stop?"=w11, "Module Admin in"=w13) -> ("error out"=w22:errorcluster, "External Launch"=w10:bool, "Module Admin out"=w12:refnum<class "Delacor_lib_QMH_Cloneable Module Admin.lvclass">)  [unwired: 6 in]
  n148 = Unregister For Events(event registration refnum=w17, error in=w22) -> (error out=w21:errorcluster)
  "error out" <- w21
  n149 = local write "Module Admin"(w12) -> ()
  n150 = case "External Launch?" shown="True" w10 {
    tunnel: w21 -> [_ w374]
    frame False {
    }
    frame True {
      n151 = case shown="No Error" w374 {
        frame No Error {
          n152 = invoke class="VI" method="FP.Close"() -> ()  [unwired: 3 in, 3 out]
        }
        frame Error {
          n153 = invoke class="VI" method="FP.Open"("Activate"=TRUE ("Activate?")) -> ()  [unwired: 4 in, 5 out]
        }
      }
    }
  }
